vi "FA_AgentConfig_Open.vi"(8 "Error In":errorcluster, 9 "Current VI Path":path, 10 "Dev":bool) -> (0 "Error Out":errorcluster, 3 "INI File Path":T1)   [LabVIEW 2013, in "FA_AgentConfig.lvlib"]
doc: "Opens the FA_Config.ini file"
uses:
  FA_AgentConfig.lvlib
  FA_AgentConfig_Refnum.ctl
  <vilib>/Utility/config.llb/Config Data RefNum.ctl
  <vilib>/Utility/config.llb/NI_LVConfig.lvlib
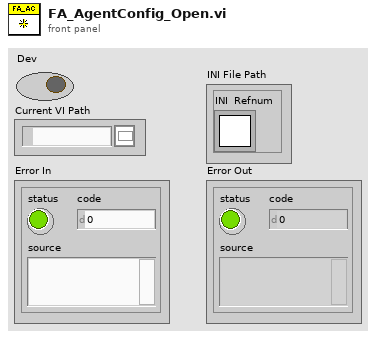
[diagram p1: front panel]
types:
  T1 = typedef "FA_AgentConfig.lvlib/FA_AgentConfig_Refnum.ctl" = cluster{"INI  Refnum":T2}
  T2 = typedef "NI_LVConfig.lvlib/Config Data RefNum.ctl" = refnum<k1>
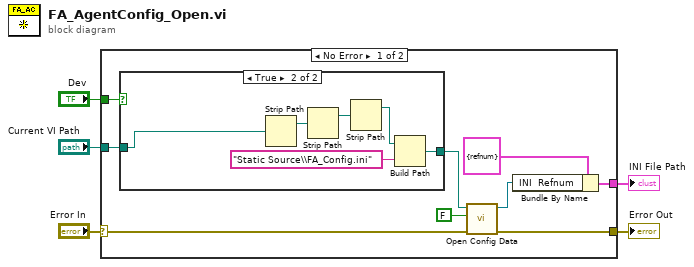
[diagram p0: block diagram]
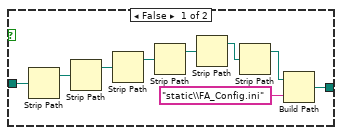
[diagram p2: hidden frame]
diagram:
  n1 = case shown="No Error" "Error In" {
    selector: "Error In" -> [w6 w30]
    tunnel: [w11 w30] -> w4
    tunnel: "Dev" -> [w14 _]
    tunnel: [w12 _] -> w2
    tunnel: "Current VI Path" -> [w7 _]
    frame No Error {
      n2 = case shown="True" w14 {
        tunnel: [w16 w29] -> w10
        tunnel: w7 -> [w15 w24]
        frame False {
          n3 = Strip Path(path=w15) -> (stripped path=w23:path)  [unwired: 1 out]
          n4 = Strip Path(path=w23) -> (stripped path=w22:path)  [unwired: 1 out]
          n5 = Strip Path(path=w22) -> (stripped path=w20:path)  [unwired: 1 out]
          n6 = Strip Path(path=w20) -> (stripped path=w19:path)  [unwired: 1 out]
          n7 = Strip Path(path=w19) -> (stripped path=w18:path)  [unwired: 1 out]
          n8 = Strip Path(path=w18) -> (stripped path=w17:path)  [unwired: 1 out]
          n9 = Build Path(base path=w17, name or relative path="static\\FA_Config.ini") -> (appended path=w16:path)
        }
        frame True {
          n10 = Strip Path(path=w24) -> (stripped path=w28:path)  [unwired: 1 out]
          n11 = Strip Path(path=w28) -> (stripped path=w27:path)  [unwired: 1 out]
          n12 = Strip Path(path=w27) -> (stripped path=w26:path)  [unwired: 1 out]
          n13 = Build Path(base path=w26, name or relative path="Static Source\\FA_Config.ini") -> (appended path=w29:path)
        }
      }
      n14 = call <vilib>:"Open Config Data.vi"("error in (no error)"=w6, "create file if necessary (T)"=FALSE, "configuration file path"=w10) -> ("error out"=w11:errorcluster, "refnum"=w9:T2)  [unwired: 6 in, 1 out]
      n15 = Bundle By Name(cluster=T1 {"INI  Refnum"=refnum} ("INI File Path 2"), "INI  Refnum"=w9) -> (w12:T1)
    }
    frame Error {
    }
  }
  "Error Out" <- w4
  "INI File Path" <- w2
